vi "Copy ECATLVProvider32 Files.vi"(8 "error in":errorcluster, 9 "Build Specification Name":string, 10 "Source Path":path, 11 "Destination Path":path) -> (0 "error out":errorcluster)   [LabVIEW 2024, in "Build VIs.lvlib"]
uses:
  Build VIs.lvlib
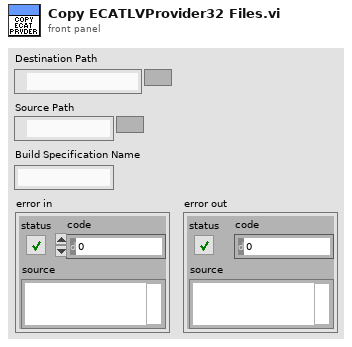
[diagram p1: front panel]
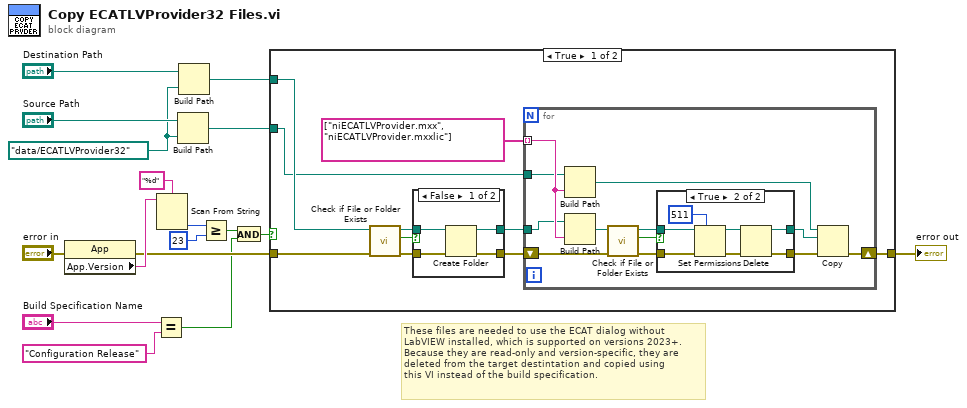
[diagram p0: block diagram]
diagram:
  w1 = path "data/ECATLVProvider32"
  # "These files are needed to use the ECAT dialog without\nLabVIEW installed, which is supported on versions 2023+.\nBecause they are read-only and version-specific, they are\ndeleted from the target destintation and copied using\nthis VI instead of the build specification."
  n1 = property class="App"(error in="error in") -> (error out=w11:errorcluster, "App.Version"=w13:string)  [unwired: 1 in, 1 out]
  n2 = Equal?(x="Build Specification Name", y="Configuration Release") -> (x = y?=w5:bool)
  n3 = Scan From String(format string="%d", input string=w13) -> (output 1=w2:i32)  [unwired: 3 in, 3 out]
  n4 = Build Path(base path="Source Path", name or relative path=w1) -> (appended path=w15:path)
  n5 = Build Path(base path="Destination Path", name or relative path=w1) -> (appended path=w10:path)
  n6 = Greater Or Equal?(x=w2, y=23) -> (x >= y?=w6:bool)
  n7 = And(x=w6, y=w5) -> (x .and. y?=w4:bool)
  n8 = case shown="True" w4 {
    tunnel: [w27 w55] -> w17
    tunnel: w15 -> [w18 _]
    tunnel: w11 -> [w20 w55]
    tunnel: w10 -> [w19 _]
    frame True {
      n9 = call <vilib>:"Check if File or Folder Exists.vi"("error in (no error)"=w20, "path"=w19) -> ("error out"=w22:errorcluster, "file or folder exists?"=w21:bool, "dup path"=w23:path)  [unwired: 7 in]
      n10 = case shown="False" w21 {
        tunnel: [w31 w33] -> w25
        tunnel: [w30 w32] -> w24
        tunnel: w23 -> [w29 w33]
        tunnel: w22 -> [w28 w32]
        frame False {
          n11 = Create Folder(path (use dialog)=w29, error in=w28) -> (created path=w31:path, error out=w30:errorcluster)  [unwired: 1 in, 1 out]
        }
        frame True {
        }
      }
      n12 = for {
        tunnel: w25 -> [w35]
        tunnel: string[] ["niECATLVProvider.mxx", "niECATLVProvider.mxxlic"] ("name or relative path") -> [w43] mode=indexing
        shift-right: [w45] -> w27
        shift-left: w24 -> [w40]
        tunnel: w18 -> [w34]
        n13 = Build Path(base path=w34, name or relative path=w43) -> (appended path=w44:path)
        n14 = Build Path(base path=w35, name or relative path=w43) -> (appended path=w38:path)
        n15 = call <vilib>:"Check if File or Folder Exists.vi"("error in (no error)"=w40, "path"=w38) -> ("error out"=w39:errorcluster, "file or folder exists?"=w36:bool, "dup path"=w37:path)  [unwired: 7 in]
        n16 = case shown="True" w36 {
          tunnel: w39 -> [w46 w51]
          tunnel: w37 -> [w47 w48]
          tunnel: [w47 w54] -> w42
          tunnel: [w46 w53] -> w41
          frame False {
          }
          frame True {
            n17 = Set Permissions(7:i16 511 ("permissions"), 8:w51, 11:w48) -> (0:w50:errorcluster, 3:w49:path)  [unwired: 2 in]
            n18 = Delete(path (use dialog)=w49, error in=w50) -> (deleted path=w54:path, error out=w53:errorcluster)  [unwired: 3 in, 1 out]
          }
        }
        n19 = Copy(8:w41, 10:w42, 11:w44) -> (0:w45:errorcluster)  [unwired: 2 in, 2 out]
      }
    }
    frame False {
    }
  }
  "error out" <- w17
